vi "CompareUnequalLength.vi"() -> ()   [LabVIEW 2013]
panel:
  out "x != y?":bool[](array[boolean])
  out "logical OR":bool
  in  "Array 2":dbl[](array[numeric])
  in  "Array":dbl[](array[numeric])
  # "INCORRECT!\n\nTry running with Array and Array2 of different lengths. Just like auto-indexing terminals on loop,\nthe result of comparing two arrays is an array of min(array1, array2)!\n\nThus, changes to elements not initialzed in other array are not flagged!"
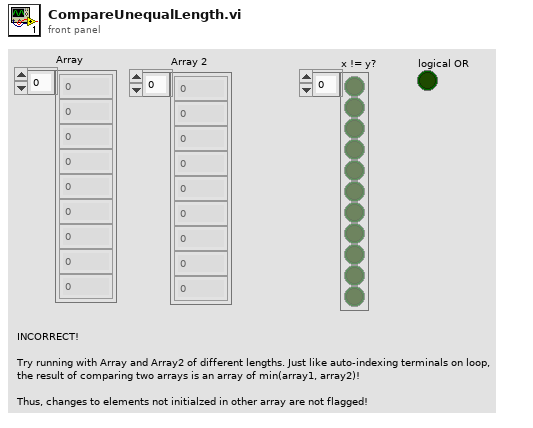
[diagram p1: front panel]
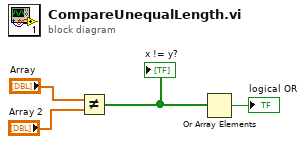
[diagram p0: block diagram]
diagram:
  n1 = Not Equal?(x="Array", y="Array 2") -> (x != y?=w2:bool[])
  "x != y?" <- w2
  n2 = Or Array Elements(Boolean array=w2) -> (logical OR=→"logical OR":bool)
